vi "Difference.vi"(7 "error in (no error)":errorcluster, 8 "Compare to this JSON Object":string="{}", 10 "JSON Object":string="{}") -> (0 "error out":errorcluster, 3 "<JSON>":string caption="<JSON>Changes")   [LabVIEW 2017, in "JSONtext.lvlib"]
doc: "Compares (\"Diffs\") a JSON Object to another JSON Object.\n\nReturns a reduced-size Object that includes only changed elements."
uses:
  JSONtext.lvlib
  <vilib>/Utility/error.llb/Error Cluster From Error Code.vi
  support/Format JSON Object.vi
  support/Format JSON Array Text.vi
  <vilib>/JDP Science/JDP Science Common Utilities/JDP Utility.lvlib
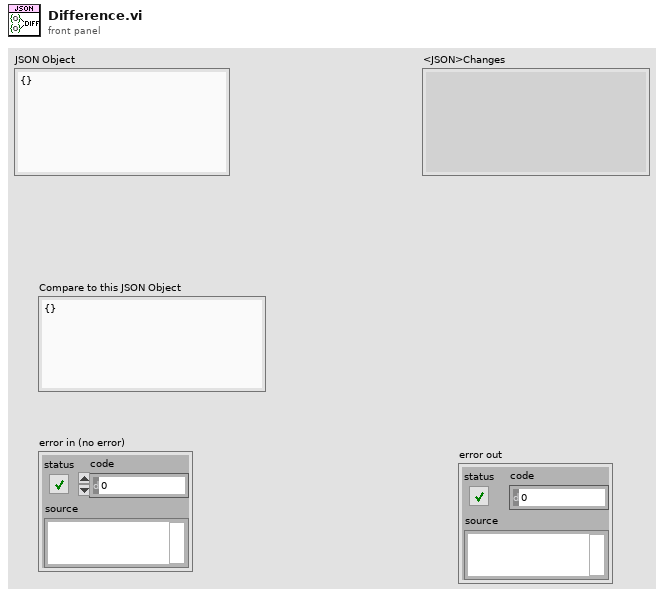
[diagram p1: front panel]
types:
  T1 = typedef "JSONtext.lvlib/JSON Value Type.ctl" = enum16{"Not a JSON Value", "JSON Object", "JSON Array", "String", "Number", "true", "false", "null"}
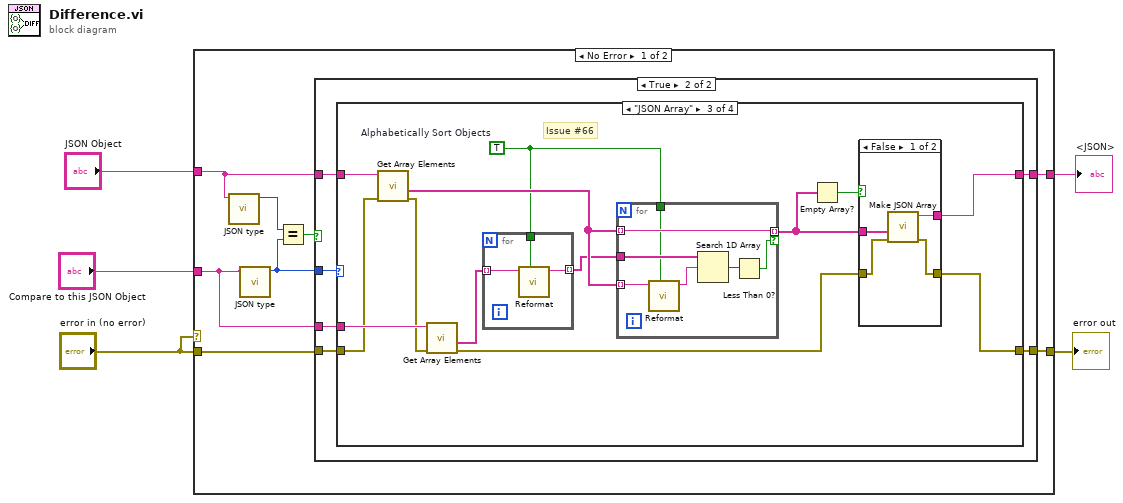
[diagram p0: block diagram]
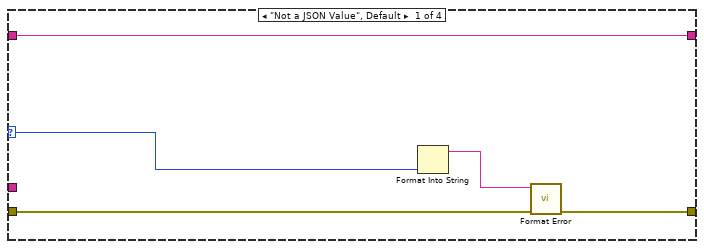
[diagram p3: hidden frame]
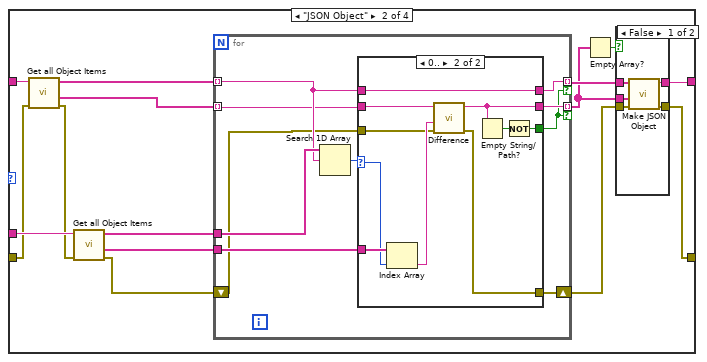
[diagram p4: hidden frame]
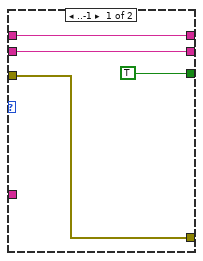
[diagram p6: hidden frame]
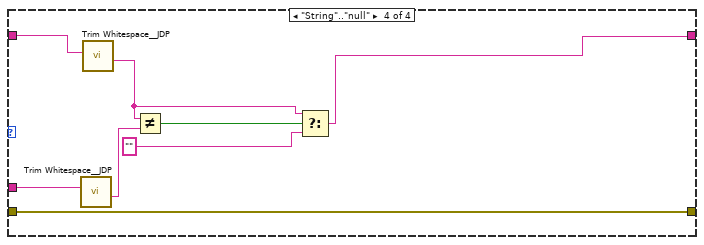
[diagram p8: hidden frame]
diagram:
  n1 = case shown="No Error" "error in (no error)" {
    tunnel: "error in (no error)" -> [w6 w108]
    tunnel: [w13 _] -> w5
    tunnel: "JSON Object" -> [w12 _]
    tunnel: "Compare to this JSON Object" -> [w11 _]
    tunnel: [w7 w108] -> w1
    frame No Error {
      n2 = call "JSON type.vi"("JSON"=w12) -> ("JSON Value Type"=w10:T1)  [unwired: 9 in, 1 out]
      n3 = call "JSON type.vi"("JSON"=w11) -> ("JSON Value Type"=w8:T1)  [unwired: 9 in, 1 out]
      n4 = Equal?(x=w10, y=w8) -> (x = y?=w9:bool)
      n5 = case shown="True" w9 {
        tunnel: w6 -> [w14 w21]
        tunnel: [w15 w20] -> w13
        tunnel: w12 -> [w15 w19]
        tunnel: w11 -> [_ w18]
        tunnel: w8 -> [_ w17]
        tunnel: [w14 w16] -> w7
        frame False {
        }
        frame True {
          n6 = case shown="\"JSON Array\"" w17 {
            selector: w17 -> [w24 _ _ _]
            tunnel: w21 -> [w22 w31 w77 w100]
            tunnel: [w26 w37 w81 w101] -> w20
            tunnel: w19 -> [w26 w36 w84 w107]
            tunnel: w18 -> [_ w35 w83 w106]
            tunnel: [w25 w27 w75 w100] -> w16
            frame "Not a JSON Value", Default {
              n7 = Format Into String(w24) -> (resulting string=w23:string)  [unwired: 3 in, 1 out]
              n8 = call "Format Error.vi"("error in (no error)"=w22, "error message"=w23) -> ("error out"=w25:errorcluster)  [unwired: 9 in]
            }
            frame "JSON Object" {
              n9 = call "Get all Object Items.vi"("error in (no error)"=w31, "JSON"=w36) -> ("error out"=w30:errorcluster, "<JSON>"=w39:string[], "Item Names"=w41:string[])  [unwired: 6 in, 1 out]
              n10 = call "Get all Object Items.vi"("error in (no error)"=w30, "JSON"=w35) -> ("error out"=w29:errorcluster, "<JSON>"=w32:string[], "Item Names"=w40:string[])  [unwired: 6 in, 1 out]
              n11 = for {
                tunnel: w41 -> [w51] mode=indexing
                tunnel: w40 -> [w57]
                tunnel: w39 -> [w50] mode=indexing
                tunnel: [w55] -> w38 mode=indexing if=w53
                tunnel: [w54] -> w34 mode=indexing if=w53
                tunnel: w32 -> [w52]
                shift-right: [w48] -> w28
                shift-left: w29 -> [w49]
                n12 = Search 1D Array(1D array=w57, element=w51) -> (index of element=w56:i32)  [unwired: 1 in]
                n13 = case shown="0.." w56 {
                  selector: w56 -> [_ w70]
                  tunnel: w51 -> [w61 w67]
                  tunnel: w50 -> [w60 w68]
                  tunnel: [w61 w67] -> w55
                  tunnel: [w60 w66] -> w54
                  tunnel: [TRUE w65] -> w53
                  tunnel: w52 -> [_ w71]
                  tunnel: w49 -> [w58 w63]
                  tunnel: [w58 w62] -> w48
                  frame ..-1 {
                  }
                  frame 0.. {
                    n14 = Index Array(array=w71, index=w70) -> (element=w69:string)
                    n15 = call "Difference.vi"("error in (no error)"=w63, "Compare to this JSON Object"=w69, "JSON Object"=w68) -> ("error out"=w62:errorcluster, "<JSON>"=w66:string)  [unwired: 6 in]
                    n16 = Empty String/Path?(string/path=w66) -> (empty?=w64:bool)
                    n17 = Not(x=w64) -> (.not. x?=w65:bool)
                  }
                }
              }
              n18 = Empty Array?(array=w34) -> (empty?=w33:bool)
              n19 = case shown="False" w33 {
                tunnel: w38 -> [w46 _]
                tunnel: [w45 _] -> w37
                tunnel: w34 -> [w44 _]
                tunnel: w28 -> [w43 w47]
                tunnel: [w42 w47] -> w27
                frame False {
                  n20 = call "Make JSON Object.vi"("error in (no error)"=w43, "JSON Items"=w44, "Item Names"=w46) -> ("error out"=w42:errorcluster, "<JSON>"=w45:string)  [unwired: 7 in]
                }
                frame True {
                }
              }
            }
            frame "JSON Array" {
              w73 = TRUE  # Alphabetically Sort Objects
              # "Issue #66"
              n21 = call "Get Array Elements.vi"("error in (no error)"=w77, "JSON"=w84) -> ("error out"=w78:errorcluster, "<JSON>"=w82:string[])  [unwired: 7 in, 1 out]
              n22 = call "Get Array Elements.vi"("error in (no error)"=w78, "JSON"=w83) -> ("error out"=w76:errorcluster, "<JSON>"=w74:string[])  [unwired: 7 in, 1 out]
              n23 = for {
                tunnel: w74 -> [w87] mode=indexing
                tunnel: [w86] -> w72 mode=indexing
                tunnel: w73 -> [w85]
                n24 = call "Reformat.vi"("Alphabetically Sort Objects"=w85, "JSON"=w87) -> ("<JSON>First JSON Value\n\n<JSON>"=w86:string)  [unwired: 6 in, 3 out]
              }
              n25 = for {
                tunnel: w72 -> [w99]
                tunnel: w82 -> [w95] mode=indexing
                tunnel: [w98] -> w80 mode=indexing if=w96
                tunnel: w82 -> [w98] mode=indexing
                tunnel: w73 -> [w93]
                n26 = call "Reformat.vi"("Alphabetically Sort Objects"=w93, "JSON"=w95) -> ("<JSON>First JSON Value\n\n<JSON>"=w94:string)  [unwired: 6 in, 3 out]
                n27 = Search 1D Array(1D array=w99, element=w94) -> (index of element=w97:i32)  [unwired: 1 in]
                n28 = Less Than 0?(x=w97) -> (x < 0?=w96:bool)
              }
              n29 = Empty Array?(array=w80) -> (empty?=w79:bool)
              n30 = case shown="False" w79 {
                tunnel: [w91 _] -> w81
                tunnel: w80 -> [w90 _]
                tunnel: w76 -> [w89 w92]
                tunnel: [w88 w92] -> w75
                frame False {
                  n31 = call "Make JSON Array.vi"("error in (no error)"=w89, "JSON Elements"=w90) -> ("error out"=w88:errorcluster, "<JSON>"=w91:string)  [unwired: 8 in]
                }
                frame True {
                }
              }
            }
            frame "String".."null" {
              n32 = call <vilib>:"Trim Whitespace__JDP.vi"("String in"=w106) -> ("String out"=w105:string)  [unwired: 6 in]
              n33 = call <vilib>:"Trim Whitespace__JDP.vi"("String in"=w107) -> ("String out"=w102:string)  [unwired: 6 in]
              n34 = Not Equal?(x=w102, y=w105) -> (x != y?=w104:bool)
              n35 = Select(t=w102, s=w104, f="") -> (s? t:f=w101:string)
            }
          }
        }
      }
    }
    frame Error {
    }
  }
  "<JSON>" <- w5
  "error out" <- w1
